vi "SaveAcquiredImageJPG.vi"(6 "File Name with Time":bool, 8 "error in":errorcluster, 9 "Index":i32, 10 "File Name":string, 11 "Folder Path":string) -> (0 "error out":errorcluster, 2 "Source Image":T1, 3 "Image Overlay":T1, 4 "return":i32)   [LabVIEW 2019]
uses:
  <vilib>/vision/Image Controls.llb/IMAQ Image.ctl
  [Global] Image.vi
  [Global] Image Overlay.vi
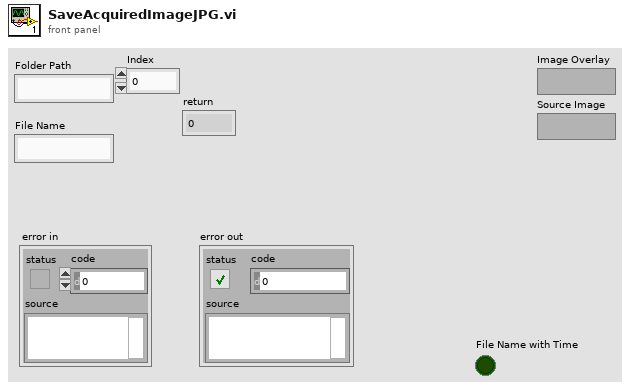
[diagram p1: front panel]
types:
  T1 = typedef "IMAQ Image.ctl" = refnum<image>
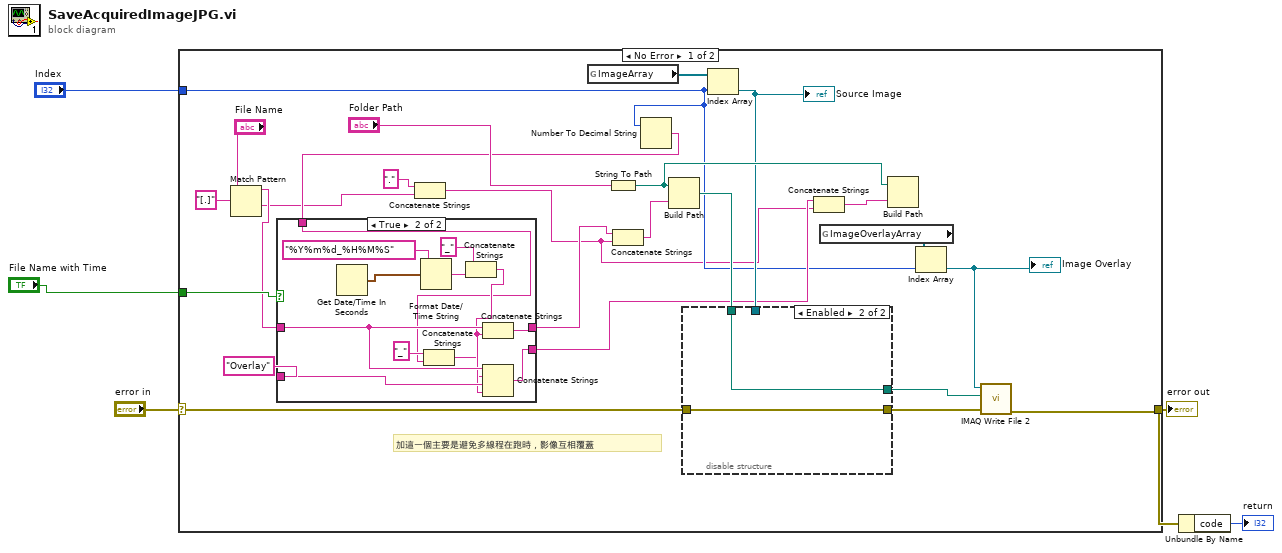
[diagram p0: block diagram]
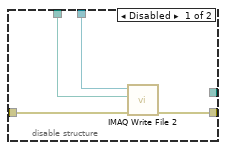
[diagram p2: hidden frame]
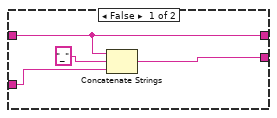
[diagram p3: hidden frame]
diagram:
  n1 = case shown="No Error" "error in" {
    selector: "error in" -> [w30 w53]
    tunnel: [w23 w53] -> w3
    tunnel: "Index" -> [w16 _]
    tunnel: "File Name with Time" -> [w20 _]
    frame No Error {
      # "加這一個主要是避免多線程在跑時，影像互相覆蓋"
      n2 = Match Pattern(string="File Name", regular expression="[.]") -> (before substring=w12:string, after substring=w11:string)  [unwired: 1 in, 2 out]
      n3 = Concatenate Strings("." ("string"), w11) -> (w9:string)
      n4 = global read "[Global] Image.vi" "ImageArray"() -> (w22:T1[])
      n5 = String To Path(string="Folder Path") -> (path=w26:path)
      n6 = Number To Decimal String(number=w16) -> (decimal integer string=w15:string)  [unwired: 1 in]
      n7 = case shown="True" w20 {
        tunnel: w12 -> [w40 w51]
        tunnel: [w40 w52] -> w19
        tunnel: [w39 w49] -> w18
        tunnel: "Overlay" ("string") -> [w38 w50]
        tunnel: w15 -> [_ w42]
        frame False {
          n8 = Concatenate Strings(w40, "_", w38) -> (w39:string)
        }
        frame True {
          n9 = Get Date/Time In Seconds() -> (seconds since 1Jan1904=w47:timestamp)
          n10 = Format Date/Time String(time format string (%c)="%Y%m%d_%H%M%S", seconds (now)=w47) -> (date/time string=w46:string)  [unwired: 1 in]
          n11 = Concatenate Strings("_", w42) -> (w41:string)
          n12 = Concatenate Strings("_" ("string"), w46) -> (w45:string)
          n13 = Concatenate Strings(w51, w45) -> (w52:string)
          n14 = Concatenate Strings(w51, w41, w50, w45) -> (w49:string)
        }
      }
      n15 = Concatenate Strings(w19, w9) -> (w28:string)
      n16 = Build Path(base path=w26, name or relative path=w28) -> (appended path=w27:path)
      n17 = Index Array(array=w22, index=w16) -> (element=w21:T1)
      "Source Image" <- w21
      n18 = disable-structure shown="Enabled" {
        disable-tunnel: w30 -> [w34 w35]
        disable-tunnel: w27 -> [w33 w36]
        disable-tunnel: [w32 w35] -> w24
        disable-tunnel: w21 -> [w31 _]
        disable-tunnel: [_ w36] -> w6
        frame Disabled {
          n19 = call-poly "IMAQ Write File 2"("error in (no error)"=w34, "File Path"=w33, "Image"=w31) -> ("error out"=w32:errorcluster)  [unwired: 7 in, 1 out]
        }
        frame Enabled {
        }
      }
      n20 = Concatenate Strings(w18, w9) -> (w25:string)
      n21 = global read "[Global] Image Overlay.vi" "ImageOverlayArray"() -> (w8:T1[])
      n22 = Build Path(base path=w26, name or relative path=w25) -> ()  [unwired: 1 out]
      n23 = Index Array(array=w8, index=w16) -> (element=w7:T1)
      "Image Overlay" <- w7
      n24 = call-poly "IMAQ Write File 2"("error in (no error)"=w24, "File Path"=w6, "Image"=w7) -> ("error out"=w23:errorcluster)  [unwired: 7 in, 1 out]
    }
    frame Error {
    }
  }
  "error out" <- w3
  n25 = Unbundle By Name(w3) -> ("code"=→"return":i32)
